vi "Get Name.vi"(8 "error in (no error)":errorcluster {"code" format="Error %.0f"}, 11 "LLB Documentation In":refnum<class "LLB Documentation.lvclass">) -> (0 "error out":errorcluster {"code" format="Error %.0f"}, 2 "Name":string, 3 "LLB Documentation Out":refnum<class "LLB Documentation.lvclass">)   [LabVIEW 2023, in "VIDoc Parsing.lvlib" / "LLB Documentation.lvclass"]
uses:
  LLB Documentation.lvclass
  LLB Documentation.lvclass/LLB Documentation.ctl
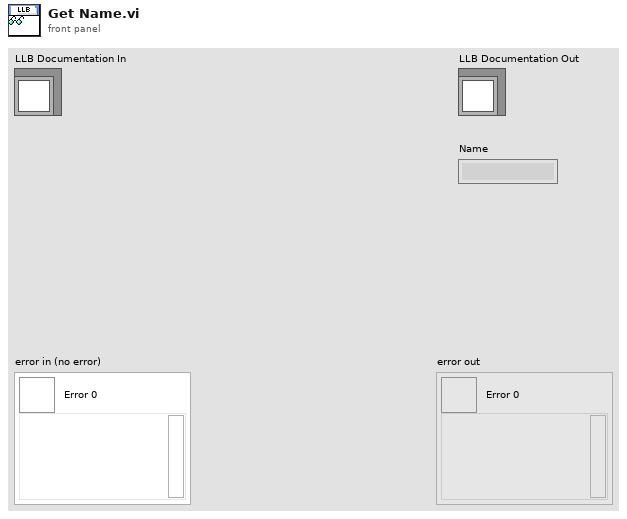
[diagram p1: front panel]
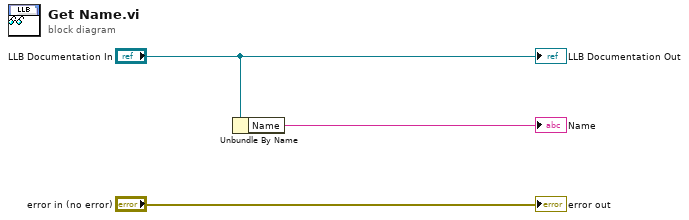
[diagram p0: block diagram]
diagram:
  n1 = Unbundle By Name("LLB Documentation In") -> ("Name"=→"Name":string)
  "error out" <- "error in (no error)"
  "LLB Documentation Out" <- "LLB Documentation In"
